vi "Write DO.vi"(8 "error in (no error)":errorcluster, 10 "Array":i32[](array[numeric]), 11 "NIDIO in":refnum<class "NIDIO.lvclass">) -> (0 "error out":errorcluster, 3 "NIDIO out":refnum<class "NIDIO.lvclass">)   [LabVIEW 2015, in "NIDIO.lvclass"]
uses:
  NIDIO.lvclass
  NIDIO.lvclass/NIDIO.ctl
  <vilib>/DAQmx/write.llb/DAQmx Write (Digital 1D U8 1Chan NSamp).vi
  <vilib>/DAQmx/miscellaneous.llb/DAQmx Fill In Error Info.vi
  DIO.lvclass
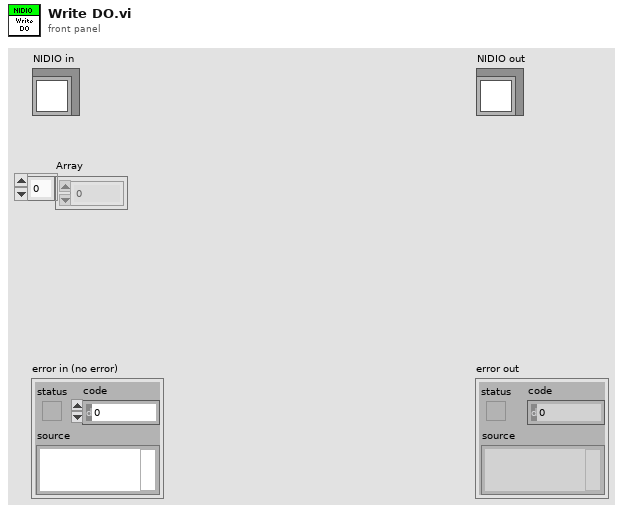
[diagram p1: front panel]
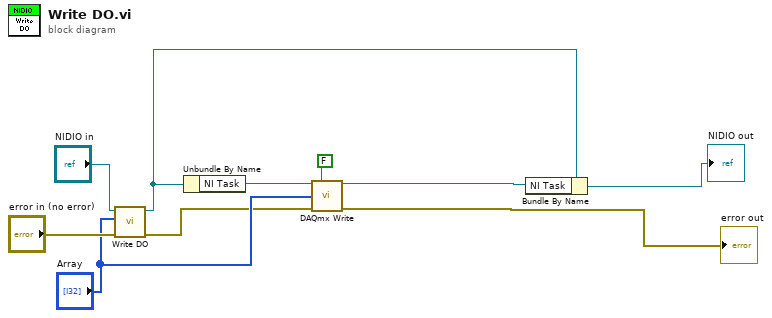
[diagram p0: block diagram]
diagram:
  n1 = call-parent "Write DO.vi"("error in (no error)"="error in (no error)", "Array"="Array", "DIO in"="NIDIO in") -> ("error out"=w5:errorcluster, "DIO out"=w4:refnum<class "NIDIO.lvclass">)  [unwired: 7 in]
  n2 = Unbundle By Name(w4) -> ("NI Task"=w7:refnum<k21>)
  n3 = call-poly <vilib>:"DAQmx Write.vi"("task/channels in"=w7, "auto start"=FALSE, "data"="Array", "error in"=w5) -> ("task out"=w1:refnum<k21>, "error out"=→"error out":errorcluster)  [unwired: 9 in, 1 out]
  n4 = Bundle By Name(cluster=w4, "NI Task"=w1) -> (→"NIDIO out":refnum<class "NIDIO.lvclass">)
